vi "Add New Or Old Port.vi"(8 "old port?":bool, 9 "refresh listbox":T1[](array[typedef]), 10 "port":T3={"hardware channel"=0, "direction"=enum."Rx", "labels"=[], "speed"=enum."HI (100 kb/s)"}) -> (1 "refresh listbox out":T1[](array[typedef]))   [LabVIEW 2024, in "AIM ARINC 429 System Explorer.lvlib" / "Implementation.lvlib"]
uses:
  Implementation.lvlib
  Types/Refresh Listbox.ctl
  Types/Refresh Symbols.ctl
  Shared/VS Channels Definition for All Labels on Hardware Channel.ctl
  Shared/Direction.ctl
  Shared/VS Channels Definition for Label.ctl
  Shared/VS Channel Definition for Parameter.ctl
  Shared/Parameter Definition.ctl
  <vilib>/NI/NI VeriStand Encoding and Decoding/Encoding.ctl
  Shared/Transfer Type.ctl
  Shared/Transfer Speed.ctl
  <vilib>/NI/NI VeriStand Encoding and Decoding/Encoding and Decoding.lvlib
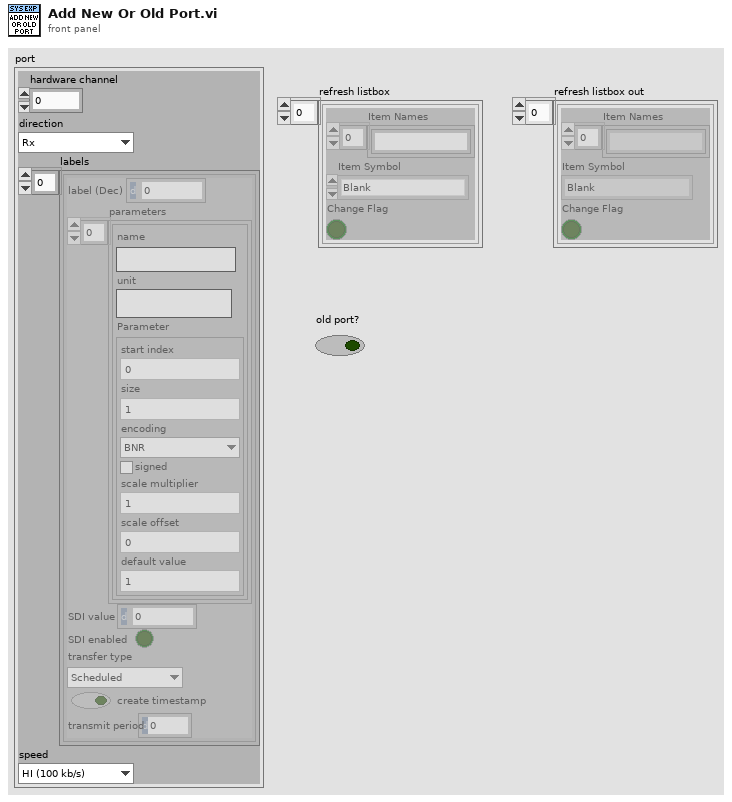
[diagram p1: front panel]
types:
  T1 = typedef "AIM ARINC 429 System Explorer.lvlib/Implementation.lvlib/Refresh Listbox.ctl" = cluster{"Item Names":string[], "Item Symbol":T2, "Change Flag":bool}
  T2 = typedef "AIM ARINC 429 System Explorer.lvlib/Implementation.lvlib/Refresh Symbols.ctl" = enum16{"Blank", "Port", "Incoming", "Outgoing", "Label", "Word", "Parameter", "ARINC-429", "Config Files", "Channel Spec", "Item"}
  T3 = typedef "VS Channels Definition for All Labels on Hardware Channel.ctl" = cluster{"hardware channel":i32, "direction":T4, "labels":T5[], "speed":T10}
  T4 = typedef "Direction.ctl" = enum16{"Rx", "Tx"}
  T5 = typedef "VS Channels Definition for Label.ctl" = cluster{"label (Dec)":u32, "parameters":T6[], "SDI value":u8, "SDI enabled":bool, "transfer type":T9, "create timestamp":bool, "transmit period":u32}
  T6 = typedef "VS Channel Definition for Parameter.ctl" = cluster{"name":string, "unit":string, "Parameter":T7}
  T7 = typedef "Parameter Definition.ctl" = cluster{"start index":i32, "size":i32, "encoding":T8, "signed":bool, "scale multiplier":dbl, "scale offset":dbl, "default value":dbl}
  T8 = typedef "Encoding and Decoding.lvlib/Encoding.ctl" = enum16{"BNR", "BCD", "Discrete"}
  T9 = typedef "Transfer Type.ctl" = enum16{"Scheduled", "Acyclic", "Block", "Strobe"}
  T10 = typedef "Transfer Speed.ctl" = enum16{"LO (12.5 kb/s)", "HI (100 kb/s)"}
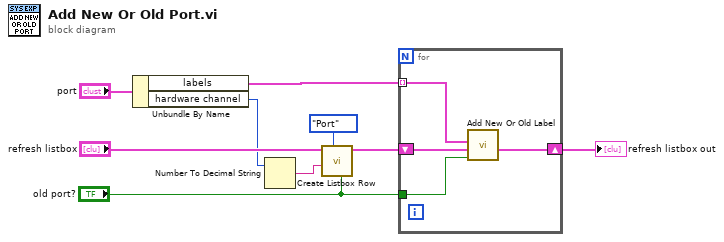
[diagram p0: block diagram]
diagram:
  n1 = Unbundle By Name("port") -> ("labels"=w5:T5[], "hardware channel"=w3:i32)
  n2 = Number To Decimal String(number=w3) -> (decimal integer string=w6:string)  [unwired: 1 in]
  n3 = call "Create Listbox Row.vi"("swap new and old (F)"="old port?", "refresh symbol (Blank)"=Refresh_Symbols."Port" ("Refresh Symbol (Blank)"), "new item"=w6, "refresh listbox"="refresh listbox") -> ("refresh listbox out"=w4:T1[])  [unwired: 7 in]
  n4 = for {
    tunnel: w5 -> [w10] mode=indexing
    shift-right: [w11] -> w1
    shift-left: w4 -> [w12]
    tunnel: "old port?" -> [w13]
    n5 = call "Add New Or Old Label.vi"("old label?"=w13, "refresh listbox"=w12, "label"=w10) -> ("refresh listbox out"=w11:T1[])  [unwired: 8 in]
  }
  "refresh listbox out" <- w1
